vi "Init Test Data Message.vi"(5 "Test Data Message":refnum<class "TestManagerMsg.Test.lvclass">, 7 "overwrite?":bool=TRUE, 9 "Test Data":T1, 10 "TestID":string, 11 "CallerID":string) -> (3 "Message":refnum<class "TestManagerMsg.lvclass">)   [LabVIEW 2020, in "Caraya.lvlib" / "TestManagerMsg.Test.lvclass"]
uses:
  TestManagerMsg.Test.lvclass
  C:/projects/caraya/src/classes/Test Manager Message/TestManagerMsg.lvclass
  Test Manager Message/TestManagerMsg.lvclass
  Test-Data -- cluster.ctl
  TestManagerMsg.Test.lvclass/TestManagerMsg.Test.ctl
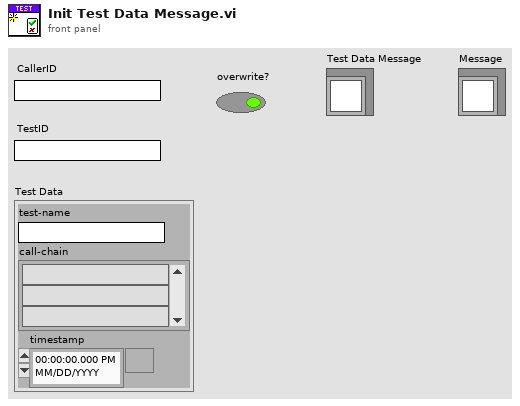
[diagram p1: front panel]
types:
  T1 = typedef "Caraya.lvlib/TestManagerMsg.Test.lvclass/Test-Data -- cluster.ctl" = cluster{"test-name":string, "call-chain":string[], "timestamp":timestamp}
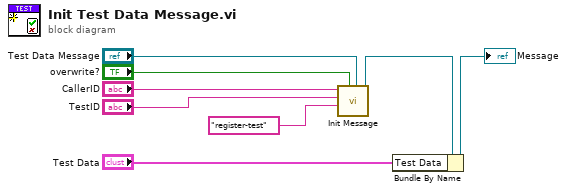
[diagram p0: block diagram]
diagram:
  n1 = call "Init Message.vi"("TestManagerMsg"="Test Data Message", "overwrite?"="overwrite?", "key"="register-test", "self-id"="TestID", "owner-id"="CallerID") -> ("Message"=w7:refnum<class "TestManagerMsg.Test.lvclass">)  [unwired: 6 in]
  n2 = Bundle By Name(cluster=w7, "Test Data"="Test Data") -> (→"Message":refnum<class "TestManagerMsg.Test.lvclass">)
